vi "Exit.vi"(8 "error in (no error)":errorcluster, 11 "Old State":refnum<class "SI_Idle.lvclass">) -> (0 "error out":errorcluster, 3 "New State":refnum<class "SI_Idle.lvclass">)   [LabVIEW 2025, in "Sensor_Iterface.lvlib" / "SI_Idle.lvclass"]
doc: "This is an abstract method. Override this method to define the behavior when you leave the state."
uses:
  SI_Idle.lvclass
  SI_Idle.lvclass/SI_Idle.ctl
  Sensor_Iterface/Sensor_Iterface.lvclass
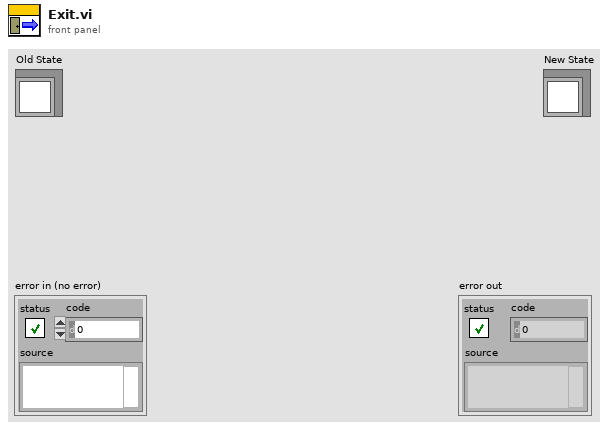
[diagram p1: front panel]
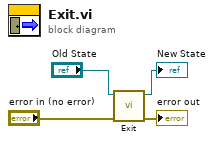
[diagram p0: block diagram]
diagram:
  n1 = call-parent "Exit.vi"("error in (no error)"="error in (no error)", "Old State"="Old State") -> ("error out"=→"error out":errorcluster, "New State"=→"New State":refnum<class "SI_Idle.lvclass">)  [unwired: 8 in]
